vi "Global Performance Test.vi"() -> ()   [LabVIEW 2021]
uses:
  Global 1.vi
panel:
  out "x-y":dbl format="%#_6p"
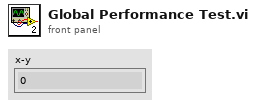
[diagram p1: front panel]
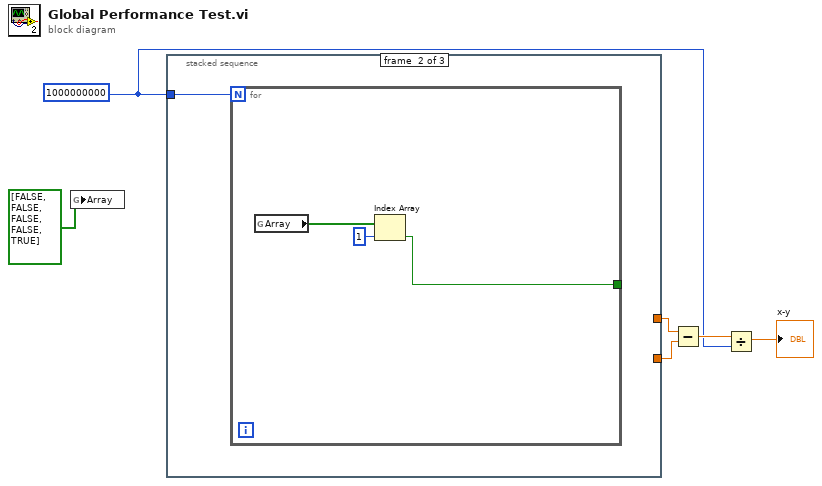
[diagram p0: block diagram]
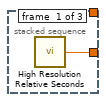
[diagram p2: hidden frame]
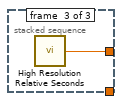
[diagram p3: hidden frame]
diagram:
  w2 = 1000000000
  n1 = global write "Global 1.vi" "Array"(bool[] [FALSE, FALSE, FALSE, FALSE, TRUE] ("Array")) -> ()
  n2 = stacked-sequence {
    tunnel: [w7 _ _] -> w6
    tunnel: [_ _ w12] -> w5
    tunnel: w2 -> [_ w8 _]
    frame #0 {
      n3 = call <vilib>:"High Resolution Relative Seconds.vi"() -> ("relative seconds"=w7:dbl)
    }
    frame #1 {
      n4 = for {
        N: w8 -> [_]
        tunnel: [w10] -> _
        n5 = global read "Global 1.vi" "Array"() -> (w11:bool[])
        n6 = Index Array(array=w11, index=1) -> (element=w10:bool)
      }
    }
    frame #2 {
      n7 = call <vilib>:"High Resolution Relative Seconds.vi"() -> ("relative seconds"=w12:dbl)
    }
  }
  n8 = Subtract(x=w5, y=w6) -> (x-y=w4:dbl)
  n9 = Divide(x=w4, y=w2) -> (x/y=→"x-y":dbl)
